vi "varXNode_Terms.vi"(1 "XRef":refnum<vi>, 2 "State In":T4) -> (0 "Terms":T1[](array[typedef]))   [LabVIEW 2020, in "varXNode.xnode"]
uses:
  <vilib>/variable/varXNode.llb/varXNode.xnode
  <vilib>/variable/varXNode.llb/varXNode.ctl
  <vilib>/variable/Type Descriptor.ctl
  <vilib>/variable/TermsTypeDef.ctl
  <vilib>/XNodeSupport/XNodeRect32.ctl
  <vilib>/XNodeSupport/XNodeInt.ctl
  <vilib>/XNodeSupport/NI_XNodeSupport.lvlib
  <vilib>/variable/NI_Variable.lvlib
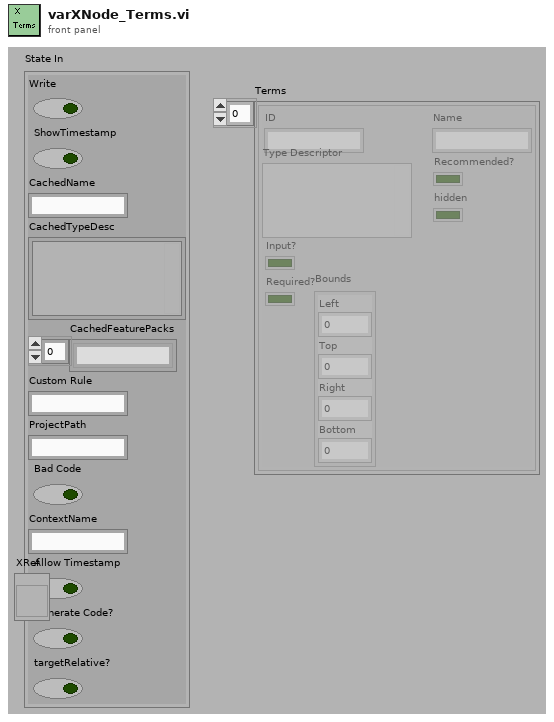
[diagram p1: front panel]
types:
  T1 = typedef "NI_Variable.lvlib/TermsTypeDef.ctl" = cluster{"ID":string, "Type Descriptor":variant, "Input?":bool, "Required?":bool, "Bounds":T2, "Name":string, "Recommended?":bool, "hidden":bool}
  T2 = typedef "NI_XNodeSupport.lvlib/XNodeRect32.ctl" = cluster{"Left":T3, "Top":T3, "Right":T3, "Bottom":T3}
  T3 = typedef "NI_XNodeSupport.lvlib/XNodeInt.ctl" = i32
  T4 = typedef "varXNode.xnode/varXNode.ctl" = cluster{"Write":bool, "ShowTimestamp":bool, "CachedName":string, "CachedTypeDesc":T5, "CachedFeaturePacks":string[], "Custom Rule":string, "ProjectPath":string, "Bad Code":bool, "ContextName":string, "Allow Timestamp":bool, "Generate Code?":bool, "targetRelative?":bool}
  T5 = typedef "NI_Variable.lvlib/Type Descriptor.ctl" = cluster{"Variant":variant}
  T6 = typedef "NI_Variable.lvlib/variable.ctl" = cluster{"Name":string, "TypeDesc":T5, "Type":string, "Typedefs":string, "Attribs":T7, "FeaturePacks":string[]}
  T7 = typedef "NI_Variable.lvlib/Attribs.ctl" = cluster{"Attrib":string, "Value":string}[]
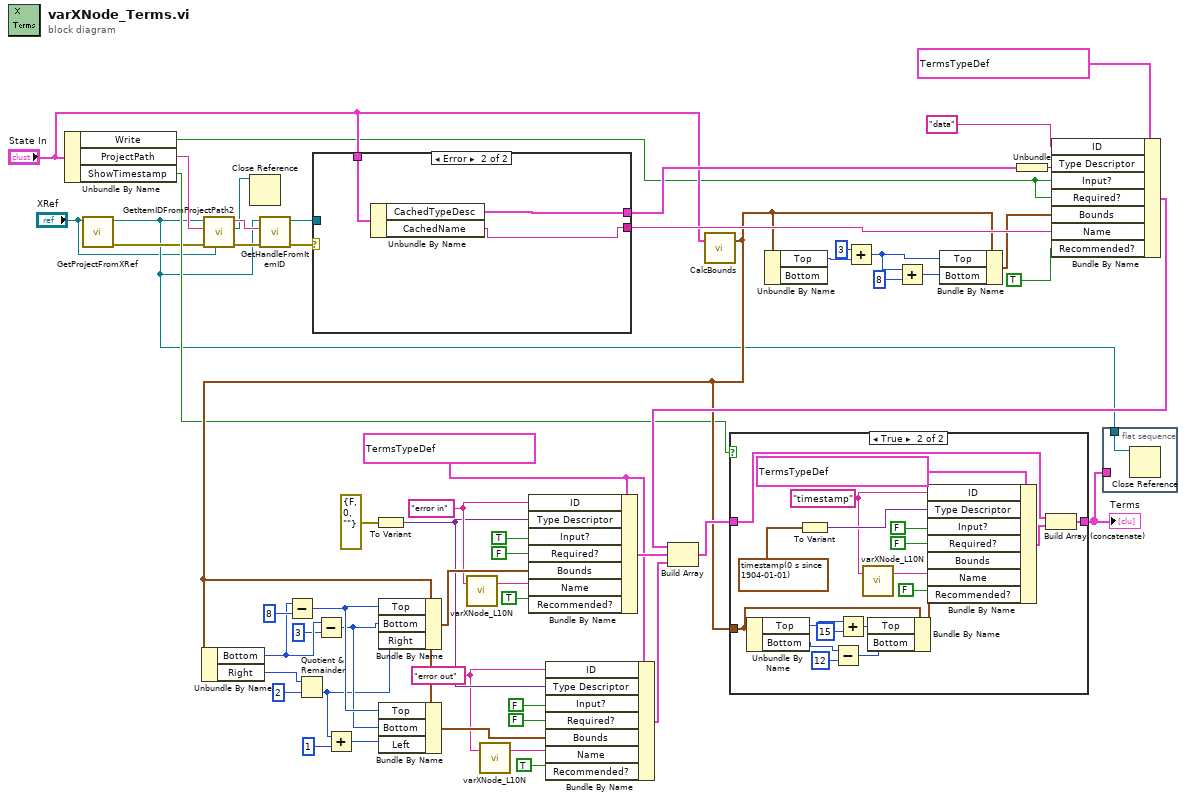
[diagram p0: block diagram]
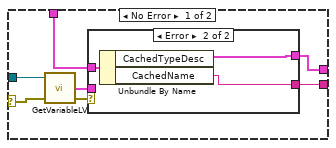
[diagram p3: hidden frame]
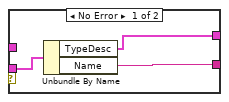
[diagram p4: hidden frame]
diagram:
  w21 = T1 {"ID"="", "Type Descriptor"=variant, "Input?"=FALSE, "Required?"=FALSE, "Bounds"={"Left"=0, "Top"=0, "Right"=0, "Bottom"=0}, "Name"="", "Recommended?"=FALSE, "hidden"=FALSE} ("Cluster")
  w5 = "error out" ("ID")
  w40 = "error in" ("ID")
  n1 = Unbundle By Name("State In") -> ("Write"=w3:bool, "ProjectPath"=w16:string, "ShowTimestamp"=w17:bool)
  n2 = call <vilib>:"GetProjectFromXRef.vi"("XRef"="XRef") -> ("error out"=w11:errorcluster, "Project"=w9:refnum<vi>)  [unwired: 9 in]
  n3 = call <vilib>:"GetItemIDFromProjectPath2.vi"("XRef"="XRef", "error in"=w11, "ProjectPath"=w16, "Project"=w9) -> ("error out"=w14:errorcluster, "ProjectItem"=w7:refnum<vi>, "Item ID"=w15:string)  [unwired: 5 in]
  n4 = Close Reference(reference=w7) -> ()  [unwired: 1 in, 1 out]
  n5 = call <vilib>:"GetHandleFromItemID.vi"("error in"=w14, "ItemID"=w15, "Project"=w9) -> ("error out"=w13:errorcluster, "VarHandle"=w12:refnum<k1>)  [unwired: 7 in]
  n6 = case shown="Error" w13 {
    selector: w13 -> [w58 _]
    tunnel: [w62 w70] -> w55
    tunnel: [w60 w69] -> w20
    tunnel: "State In" -> [w56 w71]
    tunnel: w12 -> [w59 _]
    frame No Error {
      n7 = call <vilib>:"GetVariableLV.vi"("error in"=w58, "Variable handle in"=w59) -> ("error out"=w57:errorcluster, "Variable"=w61:T6)  [unwired: 1 in, 1 out]
      n8 = case shown="Error" w57 {
        tunnel: [w65 w67] -> w62
        tunnel: w61 -> [w64 _]
        tunnel: [w63 w66] -> w60
        tunnel: w56 -> [_ w68]
        frame No Error {
          n9 = Unbundle By Name(w64) -> ("TypeDesc"=w63:T5, "Name"=w65:string)
        }
        frame Error {
          n10 = Unbundle By Name(w68) -> ("CachedTypeDesc"=w66:T5, "CachedName"=w67:string)
        }
      }
    }
    frame Error {
      n11 = Unbundle By Name(w71) -> ("CachedTypeDesc"=w69:T5, "CachedName"=w70:string)
    }
  }
  n12 = To Variant(anything=errorcluster {"status"=FALSE, "code"=0, "source"=""} ("error in")) -> (Variant=w18:variant)
  n13 = call <vilib>:"varXNode_L10N.vi"("String In"=w40) -> ("String Out"=w6:string)  [unwired: 2 in]
  n14 = call <vilib>:"varXNode_L10N.vi"("String In"=w5) -> ("String Out"=w4:string)  [unwired: 2 in]
  n15 = call <vilib>:"CalcBounds.vi"("State In"="State In") -> ("Bounds"=w22:T2)  [unwired: 2 in]
  n16 = Unbundle By Name(w22) -> ("Bottom"=w30:T3, "Right"=w26:T3)
  n17 = Subtract(x=w30, y=8 ("x")) -> (x-y=w28:T3)
  n18 = Quotient & Remainder(x=w26, y=2) -> (floor(x/y)=w24:T3)  [unwired: 1 out]
  n19 = Subtract(x=w30, y=3) -> (x-y=w27:T3)
  n20 = Add(x=w24, y=1) -> (x+y=w25:T3)
  n21 = Bundle By Name(cluster=w22, "Top"=w28, "Bottom"=w27, "Right"=w24) -> (w50:T2)
  n22 = Bundle By Name(cluster=w22, "Top"=w28, "Bottom"=w27, "Left"=w25) -> (w39:T2)
  n23 = Bundle By Name(cluster=w21, "ID"=w40, "Type Descriptor"=w18, "Input?"=TRUE, "Required?"=FALSE, "Bounds"=w50, "Name"=w6, "Recommended?"=TRUE) -> (w48:T1)
  n24 = Bundle By Name(cluster=w21, "ID"=w5, "Type Descriptor"=w18, "Input?"=FALSE, "Required?"=FALSE, "Bounds"=w39, "Name"=w4, "Recommended?"=TRUE) -> (w47:T1)
  n25 = Unbundle By Name(w22) -> ("Top"=w36:T3)  [unwired: 1 out]
  n26 = Add(x=3, y=w36) -> (x+y=w34:T3)
  n27 = Add(x=w34, y=8) -> (x+y=w32:T3)
  n28 = Bundle By Name(cluster=w22, "Top"=w34, "Bottom"=w32) -> (w37:T2)
  n29 = Unbundle(w20) -> ("Variant"=w2:variant)
  n30 = Bundle By Name(cluster=T1 {"ID"="", "Type Descriptor"=variant, "Input?"=FALSE, "Required?"=FALSE, "Bounds"={"Left"=0, "Top"=0, "Right"=0, "Bottom"=0}, "Name"="", "Recommended?"=FALSE, "hidden"=FALSE} ("Cluster"), "ID"="data", "Type Descriptor"=w2, "Input?"=w3, "Required?"=w3, "Bounds"=w37, "Name"=w55, "Recommended?"=TRUE) -> (w49:T1)
  n31 = Build Array(w49, w48, w47) -> (w51:T1[])
  n32 = case shown="True" w17 {
    tunnel: w51 -> [w72 w91]
    tunnel: [w72 w86] -> w8
    tunnel: w22 -> [_ w85]
    frame False {
    }
    frame True {
      w74 = "timestamp" ("ID")
      n33 = Unbundle By Name(w85) -> ("Top"=w84:T3, "Bottom"=w80:T3)
      n34 = To Variant(anything=timestamp(0 s since 1904-01-01) ("Time Stamp")) -> (Variant=w76:variant)
      n35 = Subtract(x=w80, y=12) -> (x-y=w79:T3)
      n36 = Add(x=w84, y=15) -> (x+y=w83:T3)
      n37 = call <vilib>:"varXNode_L10N.vi"("String In"=w74) -> ("String Out"=w73:string)  [unwired: 2 in]
      n38 = Bundle By Name(cluster=w85, "Top"=w83, "Bottom"=w79) -> (w81:T2)
      n39 = Bundle By Name(cluster=T1 {"ID"="", "Type Descriptor"=variant, "Input?"=FALSE, "Required?"=FALSE, "Bounds"={"Left"=0, "Top"=0, "Right"=0, "Bottom"=0}, "Name"="", "Recommended?"=FALSE, "hidden"=FALSE} ("Cluster"), "ID"=w74, "Type Descriptor"=w76, "Input?"=FALSE, "Required?"=FALSE, "Bounds"=w81, "Name"=w73, "Recommended?"=FALSE) -> (w90:T1)
      n40 = Build Array (concatenate)(w91, w90) -> (w86:T1[])
    }
  }
  "Terms" <- w8
  n41 = flat-sequence {
    tunnel: w9 -> [w92]
    tunnel: w8 -> [_]
    frame #0 {
      n42 = Close Reference(reference=w92) -> ()  [unwired: 1 in, 1 out]
    }
  }
